vi "Set Headers.vi"(6 "Delimiter (,)":string=",", 8 "error in (no error)":errorcluster, 9 "Update Existing? (T)":bool=TRUE, 10 "Headers[]":string[](array[string]), 11 "File Path":path) -> (0 "error out":errorcluster, 3 "File Path dup":path)   [LabVIEW 2014, in "SLL Spreadsheet.lvlib" / "SLL CSV Logger.lvclass"]
doc: "Supports writing of 2D string with new line & comma to a spreadsheet file, which are not supported by LabVIEW's builtin function.\n\nIts functionality is similar to how Excel does it - it adds double quotes to cells which contains new line character, comma and double quotes. If the cell already has double quotes, it escapes it with one more double quotes."
uses:
  SLL CSV Logger.lvclass
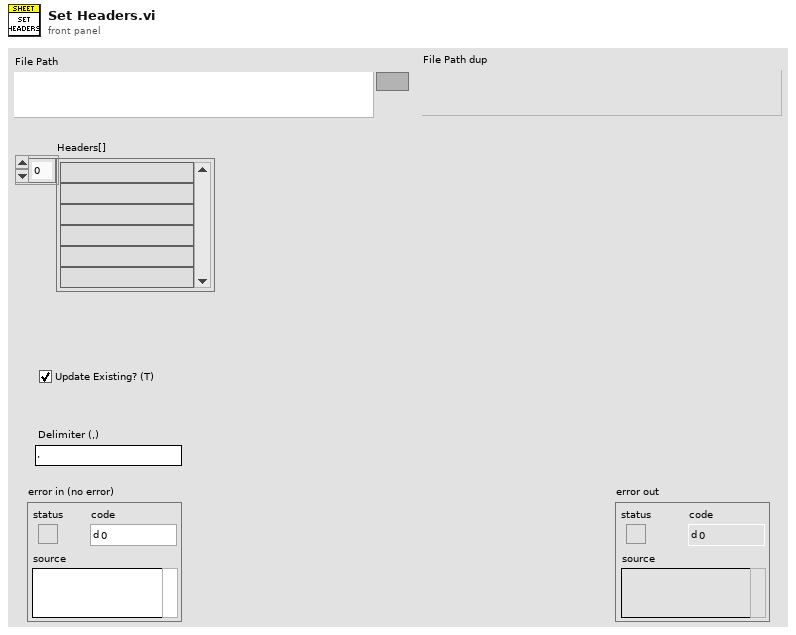
[diagram p1: front panel]
types:
  T1 = enum16{"open", "replace", "create", "open or create", "replace or create", "replace or create with confirmation"}
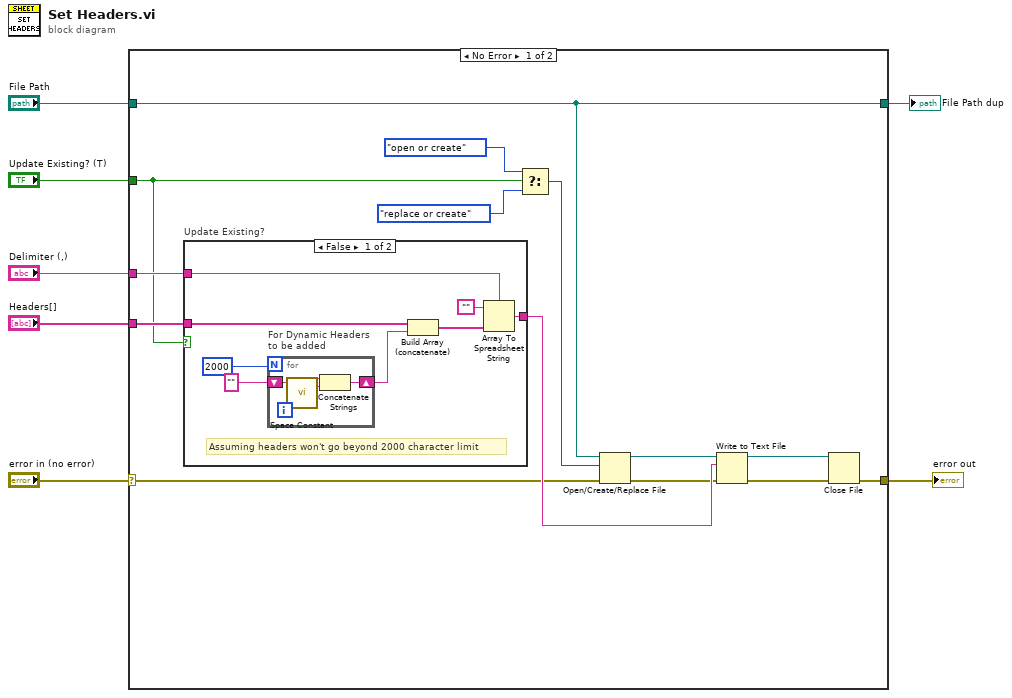
[diagram p0: block diagram]
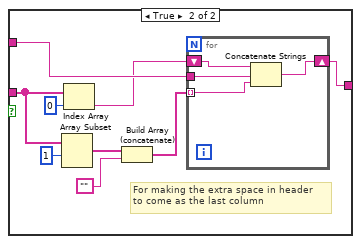
[diagram p2: hidden frame]
diagram:
  n1 = case shown="No Error" "error in (no error)" {
    selector: "error in (no error)" -> [w13 w47]
    tunnel: "Update Existing? (T)" -> [w8 _]
    tunnel: [w16 w47] -> w6
    tunnel: "Headers[]" -> [w9 _]
    tunnel: "Delimiter (,)" -> [w15 _]
    tunnel: "File Path" -> [w12 w46]
    tunnel: [w12 w46] -> w1
    frame No Error {
      n2 = case "Update Existing?" shown="False" w8 {
        tunnel: w15 -> [w29 w41]
        tunnel: [w28 w40] -> w14
        tunnel: w9 -> [w26 w37]
        frame False {
          # "Assuming headers won't go beyond 2000 character limit"
          n3 = for "For Dynamic Headers\nto be added" {
            N: 2000 -> [_]
            shift-right: [w31] -> w24
            shift-left: "" -> [w30]
            n4 = call <vilib>:"Space Constant.vi"() -> ("String"=w32:string)
            n5 = Concatenate Strings(w30, w32) -> (w31:string)
          }
          n6 = Build Array (concatenate)(w26, w24) -> (w25:string[])
          n7 = Array To Spreadsheet String(delimiter (Tab)=w29, array=w25, 3:"") -> (spreadsheet string=w28:string)
        }
        frame True {
          # "For making the extra space in header \nto come as the last column"
          n8 = Array Subset(array=w37, index=1) -> (w35:string[])  [unwired: 1 in]
          n9 = Index Array(array=w37, index=0) -> (element=w38:string)
          n10 = Build Array (concatenate)(w35, "") -> (w34:string[])
          n11 = for {
            tunnel: w34 -> [w44] mode=indexing
            tunnel: w41 -> [w45]
            shift-right: [w43] -> w40
            shift-left: w38 -> [w42]
            n12 = Concatenate Strings(w42, w45, w44) -> (w43:string)
          }
        }
      }
      n13 = Select ("function")(t=T1."open or create" ("operation (0:open)"), s=w8, f=T1."replace or create" ("operation (0:open)")) -> (s? t:f=w17:T1)
      n14 = Open/Create/Replace File(file path (use dialog)=w12, error in=w13, operation (0:open)=w17) -> (refnum out=w10:refnum<file>, error out=w11:errorcluster)  [unwired: 3 in, 1 out]
      n15 = Write to Text File(file (use dialog)=w10, text=w14, error in=w11) -> (refnum out=w19:refnum<file>, error out=w18:errorcluster)  [unwired: 1 in, 1 out]
      n16 = Close File(refnum=w19, error in=w18) -> (error out=w16:errorcluster)  [unwired: 1 out]
    }
    frame Error {
    }
  }
  "error out" <- w6
  "File Path dup" <- w1
